vi "DIAdem Parameter From Registry Get.vi"(11 "error in (no error)":errorcluster) -> (3 "DIAdem Registry Search Key":string, 4 "DIAdem Application Directory":path, 6 "DIAdem System Directory":path, 8 "DIAdem Desktop Directory":path, 10 "DIAdem Desktop File":string, 13 "DIAdem Instancing Data Type":T1(ring), 14 "DIAdem Instancing Value":u32, 15 "error out":errorcluster)   [LabVIEW 2017]
doc: "This VI reads the windows registry start parameters for DIAdem."
uses:
  <vilib>/registry/registry.llb/Registry View.ctl
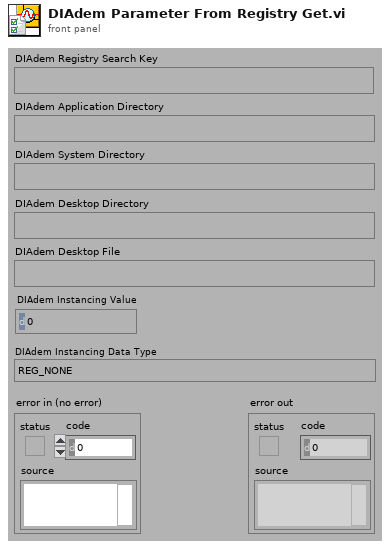
[diagram p1: front panel]
types:
  T1 = enum32{"REG_NONE", "REG_SZ", "REG_EXPAND_SZ", "REG_BINARY", "REG_DWORD_LITTLE_ENDIAN", "REG_DWORD_BIG_ENDIAN", "REG_LINK", "REG_MULTI_SZ", "REG_RESOURCE_LIST", "REG_FULL_RESOURCE_DESCRIPTOR", "REG_RESOURCE_REQUIREMENTS_LIST"}
  T2 = typedef "Registry View.ctl" = u16
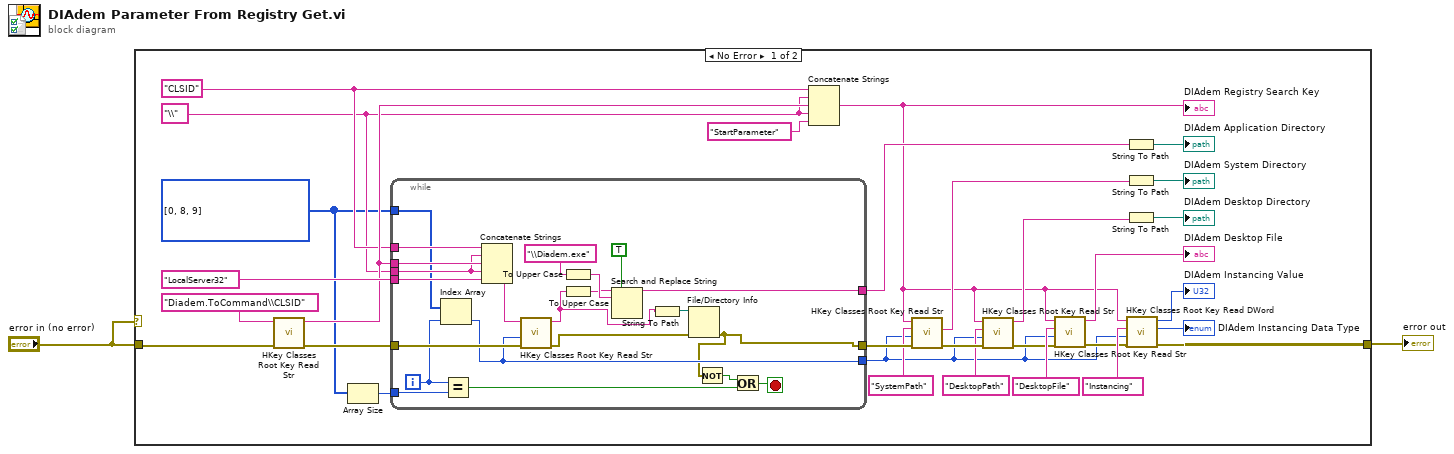
[diagram p0: block diagram]
diagram:
  n1 = case shown="No Error" "error in (no error)" {
    tunnel: "error in (no error)" -> [w29 w55]
    tunnel: [w3 w55] -> w2
    frame No Error {
      w5 = T2[] [0, 8, 9] items=["Default"=0, "KEY_WOW64_64KEY"=8, "KEY_WOW64_32KEY"=9]
      w6 = "\\" ("Substring")
      w7 = "CLSID" ("Substring")
      n2 = call <vilib>:"HKey Classes Root Key Read Str.vi"("error in (no error)"=w29, "registry search key"="Diadem.ToCommand\\CLSID" ("subkey")) -> ("error out"=w27:errorcluster, "result of registry search"=w10:string)  [unwired: 4 in]
      n3 = Array Size(array=w5) -> (size(s)=w4:i32)
      n4 = while {
        tunnel: w10 -> [w52]
        tunnel: w6 -> [w50]
        tunnel: w7 -> [w42]
        tunnel: w27 -> [w53]
        tunnel: [w34] -> w25
        tunnel: "LocalServer32" ("Substring") -> [w54]
        tunnel: [w45] -> w19
        tunnel: w5 -> [w41]
        tunnel: [w38] -> w11
        tunnel: w4 -> [w40]
        i -> [w39]
        stop <- w44 stop-if-true
        n5 = Index Array(array=w41, index=w39) -> (element=w38:T2)
        n6 = Equal?(x=w39, y=w40) -> (x = y?=w43:bool)
        n7 = Concatenate Strings(w42, w50, w52, w50, w54) -> (w51:string)
        n8 = call <vilib>:"HKey Classes Root Key Read Str.vi"("error in (no error)"=w53, "registry view"=w38, "registry search key"=w51) -> ("error out"=w35:errorcluster, "result of registry search"=w37:string)  [unwired: 3 in]
        n9 = To Upper Case(1:"\\Diadem.exe" ("search string")) -> (0:w48:string)
        n10 = To Upper Case(1:w37) -> (0:w46:string)
        n11 = Search and Replace String(replace all?=TRUE ("replace all? (F)"), input string=w46, search string=w48) -> (result string=w45:string)  [unwired: 5 in, 3 out]
        n12 = String To Path(string=w37) -> (path=w36:path)
        n13 = File/Directory Info(path=w36, error in=w35) -> (error out=w34:errorcluster)  [unwired: 6 out]
        n14 = Not(x=w34) -> (.not. x?=w33:bool)
        n15 = Or(x=w33, y=w43) -> (x .or. y?=w44:bool)
      }
      n16 = Concatenate Strings(w7, w6, w10, w6, "StartParameter" ("Substring")) -> (w9:string)
      "DIAdem Registry Search Key" <- w9
      n17 = call <vilib>:"HKey Classes Root Key Read Str.vi"("error in (no error)"=w25, "registry view"=w11, "registry search value"="SystemPath", "registry search key"=w9) -> ("error out"=w18:errorcluster, "result of registry search"=w21:string)  [unwired: 2 in]
      n18 = call <vilib>:"HKey Classes Root Key Read Str.vi"("error in (no error)"=w18, "registry view"=w11, "registry search value"="DesktopPath", "registry search key"=w9) -> ("error out"=w17:errorcluster, "result of registry search"=w14:string)  [unwired: 2 in]
      n19 = call <vilib>:"HKey Classes Root Key Read Str.vi"("error in (no error)"=w17, "registry view"=w11, "registry search value"="DesktopFile", "registry search key"=w9) -> ("error out"=w24:errorcluster, "result of registry search"=→"DIAdem Desktop File":string)  [unwired: 2 in]
      n20 = String To Path(string=w19) -> (path=→"DIAdem Application Directory":path)
      n21 = String To Path(string=w21) -> (path=→"DIAdem System Directory":path)
      n22 = String To Path(string=w14) -> (path=→"DIAdem Desktop Directory":path)
      n23 = call <vilib>:"HKey Classes Root Key Read DWord.vi"("error in (no error)"=w24, "registry view"=w11, "registry search value"="Instancing", "registry search key"=w9) -> ("error out"=w3:errorcluster, "result data type"=→"DIAdem Instancing Data Type":T1, "result of registry search"=→"DIAdem Instancing Value":u32)  [unwired: 1 in]
    }
    frame Error {
    }
  }
  "error out" <- w2
